vi "Signal+Noise.vi"() -> ()   [LabVIEW 2021]
uses:
  <vilib>/measure/NI_MABase.lvlib
panel:
  out "Waveform Graph":waveform(dbl)(graph)
  out "Baseband Signal":waveform(dbl)(graph)
  out "Noise":waveform(dbl)(graph)
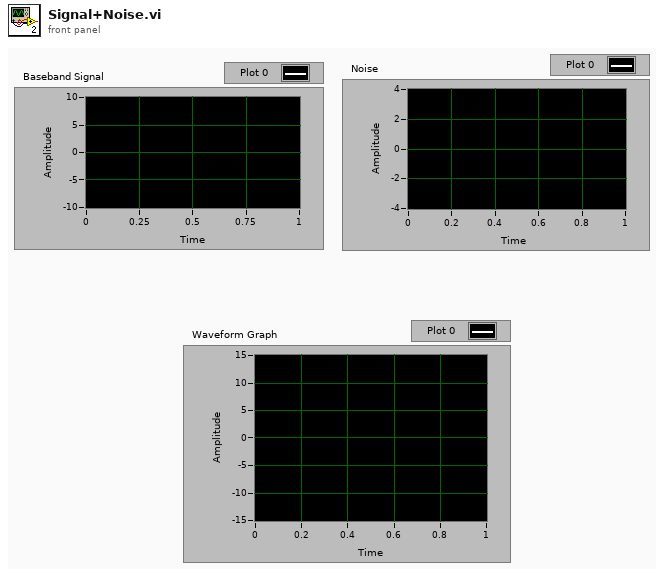
[diagram p1: front panel]
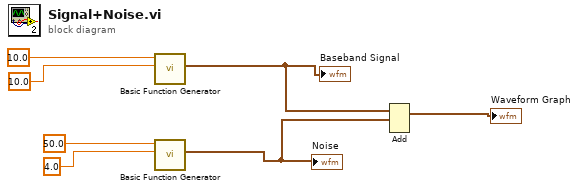
[diagram p0: block diagram]
diagram:
  n1 = call <vilib>:"Basic Function Generator.vi"("amplitude"=10.0, "frequency"=10.0) -> ("signal out"=w2:waveform(dbl))  [unwired: 7 in, 2 out]
  "Baseband Signal" <- w2
  n2 = call <vilib>:"Basic Function Generator.vi"("amplitude"=4.0, "frequency"=50.0) -> ("signal out"=w3:waveform(dbl))  [unwired: 7 in, 2 out]
  "Noise" <- w3
  n3 = Add(1:w3, 2:w2) -> (0:→"Waveform Graph":waveform(dbl))  [unwired: 1 in, 1 out]
